vi "Topmost VI who Registers all Errors.vi"() -> ()   [LabVIEW 2017]
uses:
  user.lib/_NEVSTOP/Communicable State Machine(CSM)/AdvanceAPI/CSM - Make String Arguments Safe.vi
  user.lib/_NEVSTOP/Communicable State Machine(CSM)/AdvanceAPI/CSM - Break Down Multiple States String.vi
  user.lib/_NEVSTOP/Communicable State Machine(CSM)/AdvanceAPI/CSM - Compact Multiple States.vi
  user.lib/_NEVSTOP/Communicable State Machine(CSM)/AdvanceAPI/CSM - Keywords.vi
  user.lib/_NEVSTOP/Communicable State Machine(CSM)/Communicable State Machine.lvlib
panel:
  out "State History":string
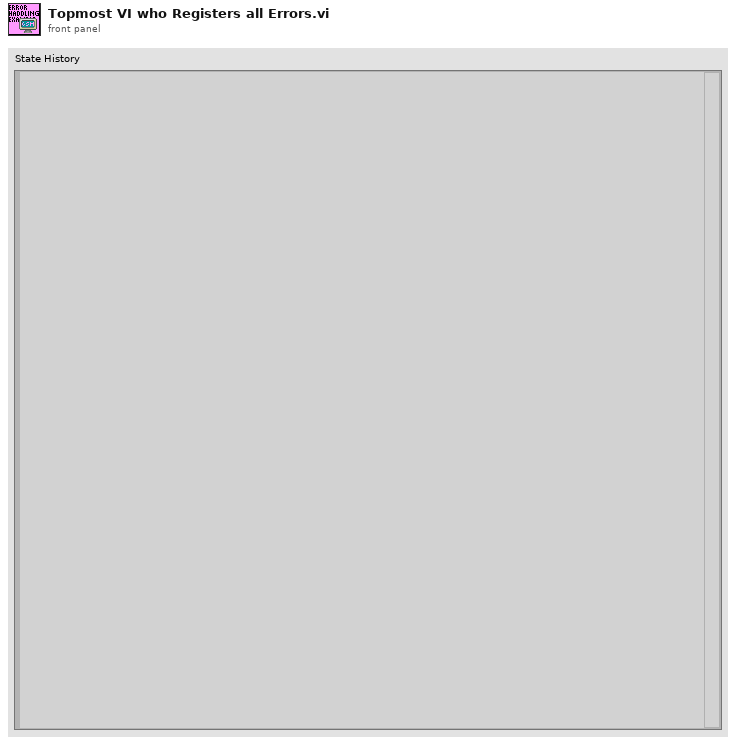
[diagram p1: front panel]
types:
  T1 = enum32{"Invalid", "Standard", "Closed", "Hidden", "Minimized", "Maximized"}
  T2 = enum32{"invalid app kind", "Development System", "Run Time System", "Student Edition", "Embedded LabVIEW", "Evaluation", "Custom"}
  T3 = typedef "Communicable State Machine.lvlib/_CSM_Response Source Message.ctl" = cluster{"‘State":string, "’Arguments":string, "’Error":errorcluster}
  T4 = cluster{"Current VI Reference":refnum<vi>, "Close Panel on Exit?":bool}
  T5 = cluster{"Core":cluster{"Current VI Reference":refnum<vi>, "Close Panel on Exit?":bool}, "Your Boolean data":bool, "Your string data":string}
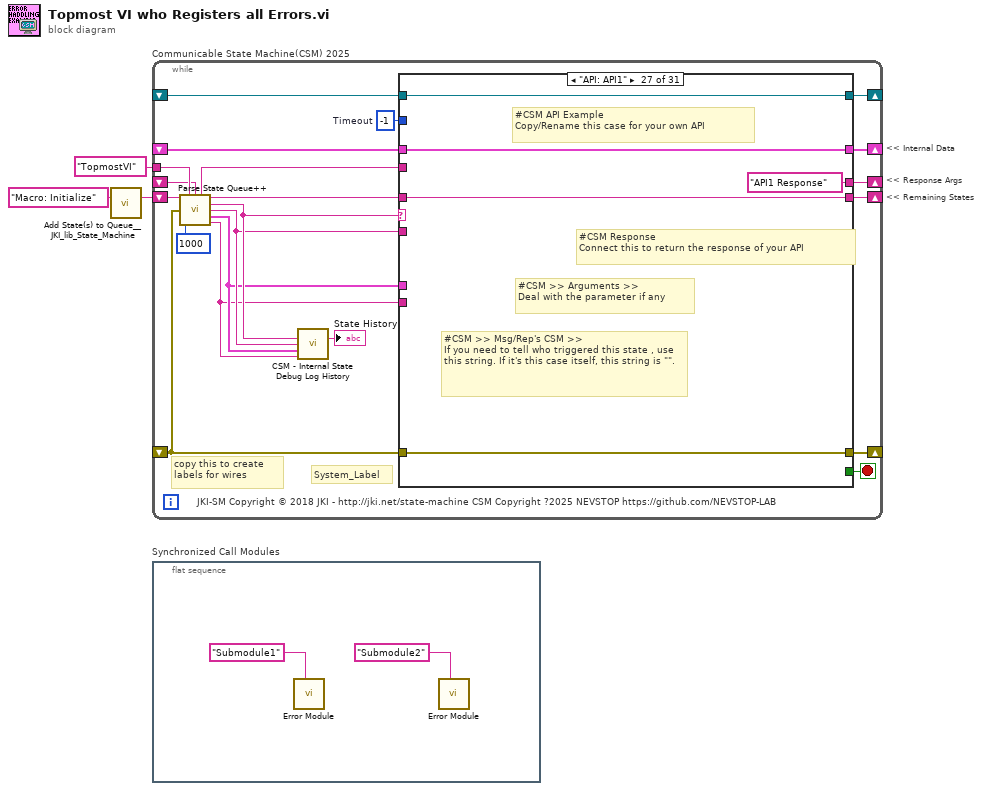
[diagram p0: block diagram]
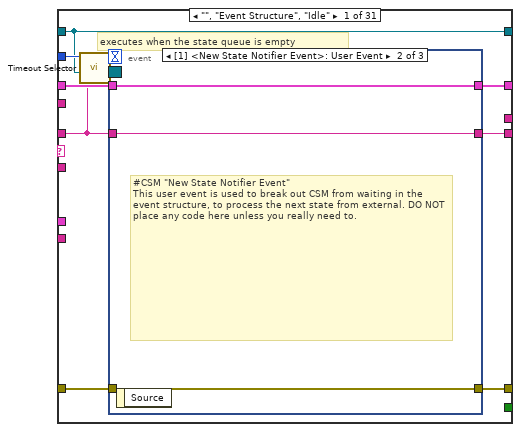
[diagram p2: hidden frame]
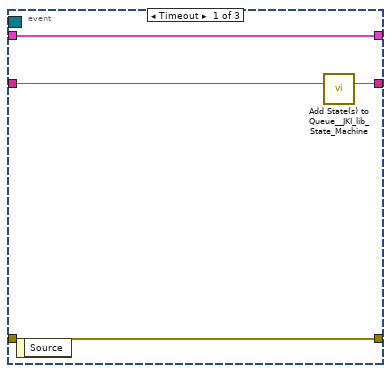
[diagram p3: hidden frame]
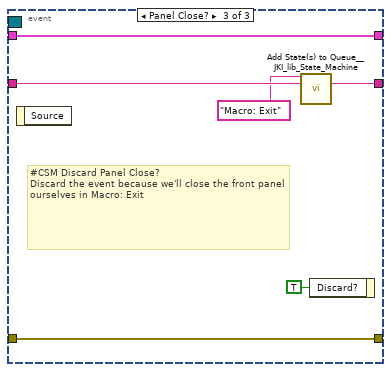
[diagram p4: hidden frame]
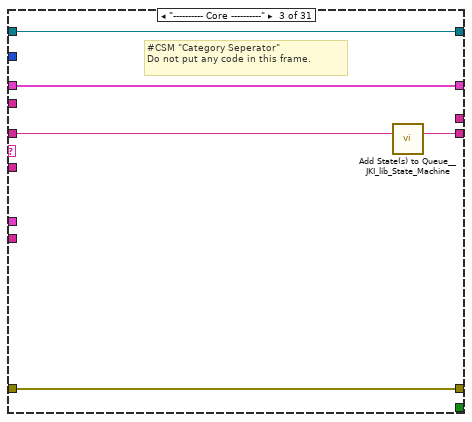
[diagram p6: hidden frame]
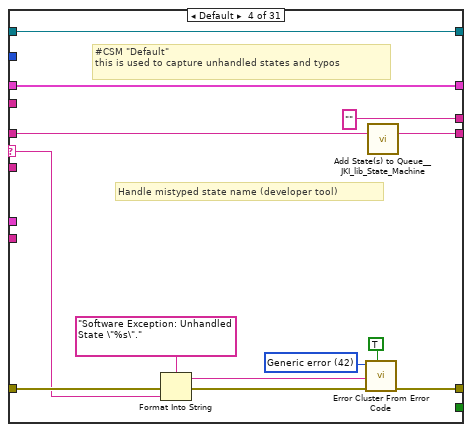
[diagram p7: hidden frame]
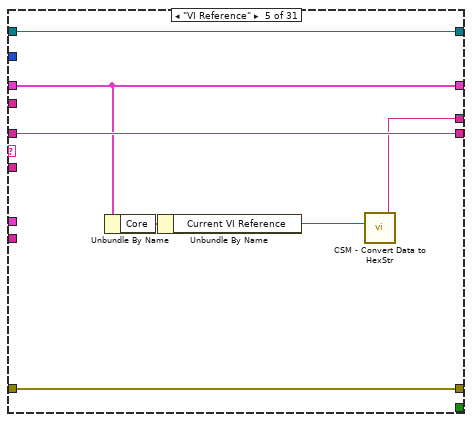
[diagram p8: hidden frame]
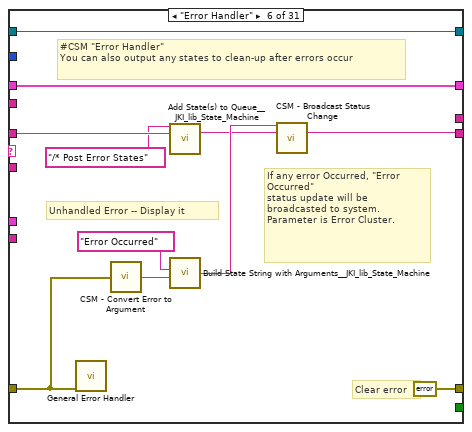
[diagram p9: hidden frame]
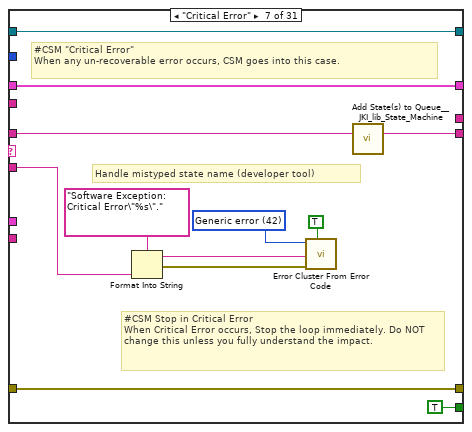
[diagram p10: hidden frame]
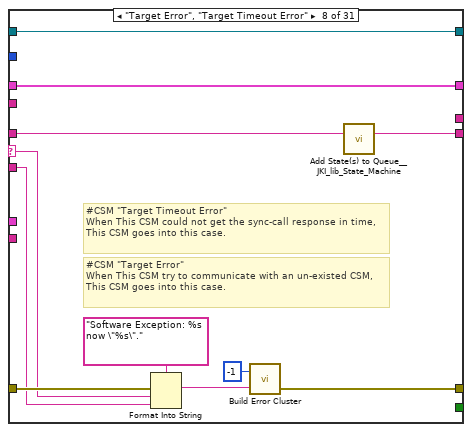
[diagram p11: hidden frame]
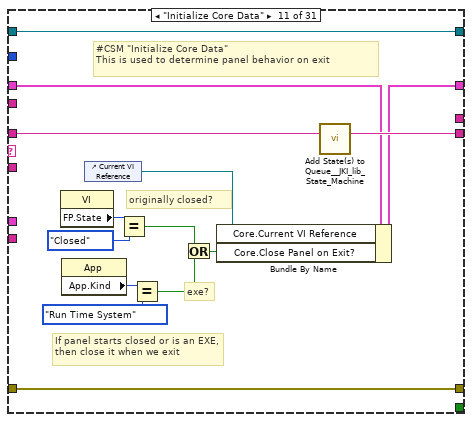
[diagram p14: hidden frame]
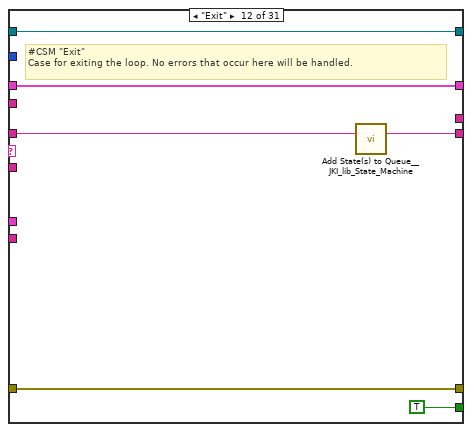
[diagram p15: hidden frame]
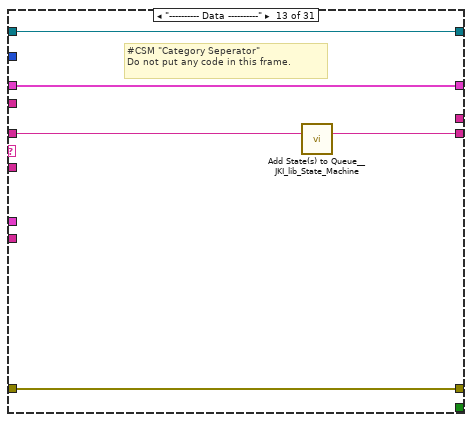
[diagram p16: hidden frame]
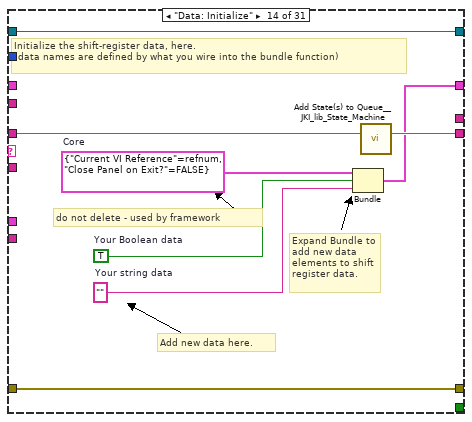
[diagram p17: hidden frame]
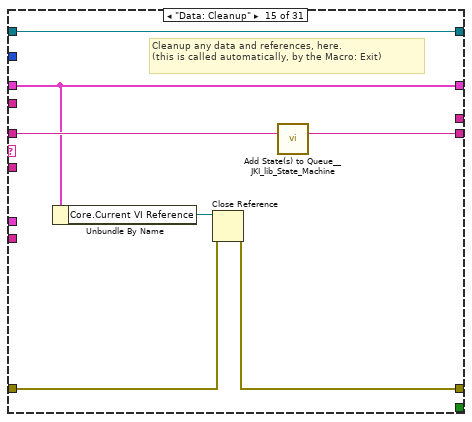
[diagram p18: hidden frame]
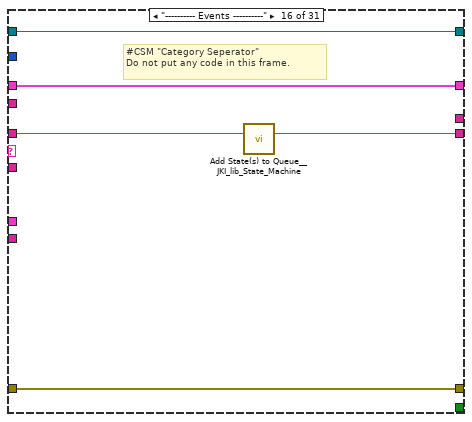
[diagram p19: hidden frame]
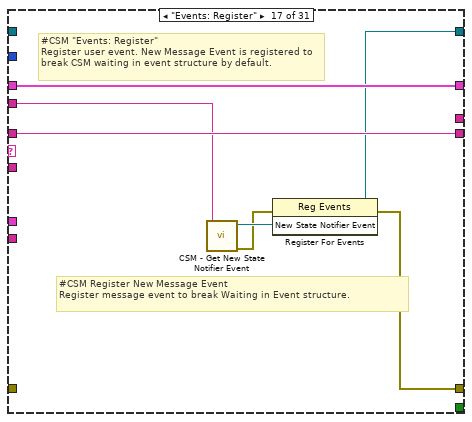
[diagram p20: hidden frame]
diagram:
  # "<< Internal Data"
  # "<< Response Args"
  # "<< Remaining States"
  n1 = call <vilib>:"Add State(s) to Queue__JKI_lib_State_Machine.vi"("State(s) in (\"\")"="Macro: Initialize") -> ("States Out"=w1:string)  [unwired: 14 in]
  n2 = while "Communicable State Machine(CSM) 2025" {
    shift-right: [w19] -> _
    shift-left: _ -> [w18]
    shift-right: [w22] -> _
    shift-left: _ -> [w16]
    shift-right: [w21] -> _
    shift-left: w1 -> [w23]
    tunnel: "TopmostVI" ("Name(\"\" to use uuid)") -> [w11]
    shift-right: [w14] -> _
    shift-left: _ -> [w5]
    shift-right: [w13] -> _
    shift-left: _ -> [w12]
    stop <- w20 stop-if-true
    w17 = -1  # Timeout
    # "copy this to create labels for wires"
    # "System_Label"
    # "JKI-SM Copyright © 2018 JKI - http://jki.net/state-machine CSM Copyright ?2025 NEVSTOP https://github.com/NEVSTOP-LAB"
    n3 = call "Parse State Queue++.vi"("State Queue"=w23, "Name(\"\" to use uuid)"=w11, "Response Arguments"=w5, "Previous Error"=w16, "Response Timeout(-2 use global Settings)"=1000 ("Response Timeout(1000ms)")) -> ("Name Used"=w6:string, "Remaining States"=w24:string, "Current State"=w10:string, "Arguments"=w9:string, ">> Response Source Message >>"=w8:T3, ">> Source CSM >>"=w7:string)  [unwired: 5 in]
    n4 = call "CSM - Internal State Debug Log History.vi"("State"=w10, "Arguments (\"\")"=w9, ">> Response Source Message >>"=w8, "Source (\"\")"=w7) -> ("Debug Log"=→"State History":string)  [unwired: 11 in]
    n5 = case shown="\"API: API1\"" w10 {
      selector: w10 -> [_ _ _ w58 _ _ _ w102 _ _ _ _ _ _ _ _ _ _ _ _ _ _ _ _ _ _ _ _ _ _ _]
      tunnel: w24 -> [w25 w49 w55 w62 w74 w86 w96 w104 w112 w116 w131 w137 w142 w150 w157 w162 w169 w173 w179 w184 w191 w207 w277 w283 w295 w298 w303 w309 w317 w323 w329]
      tunnel: w9 -> [_ _ _ _ _ _ w89 w103 _ _ _ _ _ _ _ _ _ _ _ _ w186 w201 _ _ _ _ _ w306 _ _ _]
      tunnel: w18 -> [w32 w48 w52 w60 w73 w84 w97 w106 w111 w115 w124 w135 w139 _ w152 w159 w168 w172 w176 w182 w189 w203 w274 w280 w292 w297 w302 w308 w314 w320 w326]
      tunnel: [w31 w50 w53 w64 w75 errorcluster {"status"=FALSE, "code"=0, "source"=""} ("error out") w98 w100 w113 w117 w128 w134 w140 w147 w153 w160 w163 w171 w177 w181 w187 w204 w275 w281 w293 w299 w304 w310 w315 w321 w327] -> w22
      tunnel: w16 -> [w30 w50 w53 w63 w75 w76 w98 w108 w113 w117 w128 w134 w140 w147 w154 w160 _ w174 w177 w181 w188 w205 w275 w281 w293 w299 w304 w310 w315 w321 w327]
      tunnel: [w33 w49 w54 w61 w74 w77 w95 w107 w112 w116 w130 w136 w141 w149 w156 w161 w169 w173 w178 w183 w190 w206 w276 w282 w294 w298 w303 w309 w316 w322 w328] -> w21
      tunnel: [_ _ _ _ _ _ TRUE _ _ _ _ TRUE _ _ _ _ _ _ _ _ _ _ _ _ _ _ _ _ _ _ _] -> w20
      tunnel: [w29 w48 w52 w60 w73 w84 w97 w106 w111 w115 w129 w135 w139 w148 w152 w159 w168 w172 w176 w182 w189 w203 w274 w280 w292 w297 w302 w308 w314 w320 w326] -> w19
      tunnel: w17 -> [w28 _ _ _ _ _ _ _ _ _ _ _ _ _ _ _ _ _ _ _ _ _ _ _ _ _ _ _ _ _ _]
      tunnel: w7 -> [_ _ _ _ _ _ _ _ _ _ _ _ _ _ _ _ _ _ _ _ _ _ _ _ _ _ _ _ _ _ _]
      tunnel: w8 -> [_ _ _ _ _ _ _ _ _ _ _ _ _ _ _ _ _ _ _ _ _ _ _ _ _ _ _ _ _ _ _]
      tunnel: [_ _ _ "" w69 _ _ _ _ _ _ _ _ _ _ _ _ _ _ _ _ _ _ _ _ _ "API1 Response" w305 _ "DoA Finished" "DoB Finished"] -> w14
      tunnel: [w27 w47 w51 w56 w72 w82 w87 w105 w110 w114 w118 w132 w138 w143 w151 w158 w167 w170 w175 w180 w185 w200 w273 w278 w285 w296 w301 w307 w313 w319 w325] -> w13
      tunnel: w12 -> [w27 w47 w51 w56 w72 w82 w87 w105 w110 w114 w118 w132 w138 w143 w151 w158 _ w170 w175 w180 w185 w200 w273 w278 w285 w296 w301 w307 w313 w319 w325]
      tunnel: w6 -> [_ _ _ _ _ _ _ _ _ _ _ _ _ _ _ _ w166 _ _ _ _ _ _ _ _ _ _ _ _ _ _]
      frame "", "Event Structure", "Idle" {
        # "executes when the state queue is empty"
        n6 = call "Timeout Selector.vi"("Remaining States"=w25, "Timeout Expected"=w28) -> ("Timeout"=w26:i32)  [unwired: 5 in]
        n7 = event shown="[1] <New State Notifier Event>: User Event" {
          selector: w27 -> [_ _ _]
          dyn-events: _ -> [_ _ _]
          timeout: w26 -> [_ _ _]
          tunnel: w25 -> [w37 w39 w46]
          tunnel: [w36 w39 w45] -> w33
          tunnel: w32 -> [w34 w40 w43]
          tunnel: [w35 w38 w44] -> w31
          tunnel: w30 -> [w35 w38 w44]
          tunnel: [w34 w40 w43] -> w29
          event Timeout {
            n8 = event-data() -> ()  [unwired: 1 in, 1 out]
            n9 = call <vilib>:"Add State(s) to Queue__JKI_lib_State_Machine.vi"("State(s) in (\"\")"=w37) -> ("States Out"=w36:string)  [unwired: 14 in]
          }
          event User Event {
            # "#CSM \"New State Notifier Event\"\nThis user event is used to break out CSM from waiting in the event structure, to process the next state from external. DO NOT place any code here unless you really need to."
            n10 = event-data() -> ()  [unwired: 1 in, 1 out]
          }
          event Panel Close? {
            # "#CSM Discard Panel Close?\nDiscard the event because we'll close the front panel ourselves in Macro: Exit"
            n11 = event-data() -> ()  [unwired: 1 in, 1 out]
            n12 = call <vilib>:"Add State(s) to Queue__JKI_lib_State_Machine.vi"("State(s) in Front (\"\")"="Macro: Exit", "State(s) in (\"\")"=w46) -> ("States Out"=w45:string)  [unwired: 13 in]
            n13 = event-data("Discard?"=TRUE) -> ()  [unwired: 1 in, 1 out]
          }
        }
      }
      frame "CSM Documentation" {
        # "#CSM README FIRST\n\nCSM is a LabVIEW application framework that builds upon JKI State Machine (JKISM). It follows the pattern of JKISM and extends the keywords to describe message communication between CSM modules, including concepts such as Sync-Message, Async-Message, Subscription/Unsubscription of status - essential elements for creating reusable code modules. For more information, please visit the CSM wiki: https://github.com/NEVSTOP-LAB/JKI-State-Machine-Plus-Plus/wiki\n\nFor instructions on JKI State Machine, visit: http://jki.net/state-machine/\nFor information about CSM, visit: https://github.com/NEVSTOP-LAB"
        # "#CSM \"Documentation\"\nCase for holding CSM Documenation"
      }
      frame "---------- Core ----------" {
        # "#CSM \"Category Seperator\"\nDo not put any code in this frame."
        n14 = call <vilib>:"Add State(s) to Queue__JKI_lib_State_Machine.vi"("State(s) in (\"\")"=w55) -> ("States Out"=w54:string)  [unwired: 14 in]
      }
      frame Default {
        w67 = 42 items=["No error", "Argument error", "Memory is full", "Out of zone", "End of file", "File already open", "Generic file I/O error", "File not found", "File permission error", "Disk is full", "Duplicate path", "Too many files open", "System feature not enabled", "Resource file not found", "Cannot add resource", "Resource not found", "Image not found", "Image memory error", "Pen does not exist", "Config type invalid", "Config token not found", "Config parse error", "Config memory error", "Bad external code format", "Bad external code offset", "External code not present", "Null window", "Destroy window error", "Null menu", "Print aborted", "Bad print record", "Print driver error", "Windows error during printing", "Memory error during printing", "Print dialog error", "Generic print error", "Invalid device refnum", "Device not found", "Device parameter error", "Device unit error", "Cannot open device", "Device call aborted", "Generic error", "Cancelled by user", "Object ID too low", "Object ID too high", "Object not in heap", "Unknown heap", "Unknown object (invalid DefProc)", "Unknown object (DefProc not in table)", "Message out of range", "Invalid (null) method", "Unknown message", "Manager call not supported", "Bad address", "Network operation in progress", "Network operation timed out", "Connection is busy", "Network attribute not supported", "Network error", "Address in use", "System out of memory", "Connection aborted", "Connection refused", "Not connected", "Already connected", "Connection closed", "Initialization error (interapplication manager)", "Bad occurrence", "Wait on unbound occurrence handler", "Occurrence queue overflow", "Datalog type conflict", "Unused", "Unrecognized type (interapplication manager)", "Memory corrupt", "Failed to make temporary DLL", "Old CIN version", "Drag socket not found", "Failed to load drop-object", "Failed to register OLE object", "Failed to release OLE object", "Format specifier type mismatch", "Unknown format specifier", "Too few format specifiers", "Too many format specifiers", "Scan failed", "Newer CIN version", "Error converting to variant", "Runtime menu error", "Password tampered", "Variant attribute not found", "Incompatible variant data type", "Event data is not available", "Event Store is not present", "Occurrence is not found", "Event Queue is not created", "Event info is not available", "Refnum passed is NULL", "Error retrieving Class GUID", "Error retrieving CoClass GUID", "Error retrieving TypeLib GUID.", "Bad built application magic bytes.", "Specific driver is different from the specific driver associated with the Logical Name.", "There is no session opened to the class driver.", "Max Error", "MAX - Error with config objects", "MAX - Error loading configuration", "MAX - Group not supported"]
        # "#CSM \"Default\"\nthis is used to capture unhandled states and typos"
        # "Handle mistyped state name (developer tool)"
        n15 = Format Into String(format string="Software Exception: Unhandled State \"%s\"." ("message"), error in=w63, w58) -> (resulting string=w66:string, error out=w65:errorcluster)  [unwired: 1 in]
        n16 = call <vilib>:"Error Cluster From Error Code.vi"("show call chain? (False)"=TRUE, "error in (no error)"=w65, "error message (\"\")"=w66, "error code (0)"=w67) -> ("error out"=w64:errorcluster)  [unwired: 5 in]
        n17 = call <vilib>:"Add State(s) to Queue__JKI_lib_State_Machine.vi"("State(s) in (\"\")"=w62) -> ("States Out"=w61:string)  [unwired: 14 in]
      }
      frame "VI Reference" {
        n18 = Unbundle By Name(w73) -> ("Core"=w71:T4)
        n19 = Unbundle By Name(w71) -> ("Current VI Reference"=w70:refnum<vi>)
        n20 = call "CSM - Convert Data to HexStr.vi"("Variant"=w70) -> ("HEX String (0-9,A-F)"=w69:string)  [unwired: 8 in]
      }
      frame "Error Handler" {
        # "#CSM \"Error Handler\"\nYou can also output any states to clean-up after errors occur"
        # "If any error Occurred, \"Error Occurred\" \nstatus update will be broadcasted to system.\nParameter is Error Cluster."
        # "Unhandled Error -- Display it"
        # "Clear error"
        n21 = call <vilib>:"General Error Handler.vi"("error in (no error)"=w76) -> ()  [unwired: 10 in, 5 out]
        n22 = call "CSM - Convert Error to Argument.vi"("error"=w76) -> ("Argument"=w80:string)  [unwired: 4 in]
        n23 = call <vilib>:"Add State(s) to Queue__JKI_lib_State_Machine.vi"("State(s) in Front (\"\")"="/* Post Error States", "State(s) in (\"\")"=w86) -> ("States Out"=w78:string)  [unwired: 13 in]
        n24 = call <vilib>:"Build State String with Arguments__JKI_lib_State_Machine.vi"("Arguments (\"\")"=w80, "State"="Error Occurred" ("Status with Arguments")) -> ("State with Arguments"=w79:string)  [unwired: 4 in]
        n25 = call "CSM - Broadcast Status Change.vi"("Status with Arguments"=w79, "State Queue"=w78) -> ("Remaining States"=w77:string)  [unwired: 13 in]
      }
      frame "Critical Error" {
        w93 = 42 items=["No error", "Argument error", "Memory is full", "Out of zone", "End of file", "File already open", "Generic file I/O error", "File not found", "File permission error", "Disk is full", "Duplicate path", "Too many files open", "System feature not enabled", "Resource file not found", "Cannot add resource", "Resource not found", "Image not found", "Image memory error", "Pen does not exist", "Config type invalid", "Config token not found", "Config parse error", "Config memory error", "Bad external code format", "Bad external code offset", "External code not present", "Null window", "Destroy window error", "Null menu", "Print aborted", "Bad print record", "Print driver error", "Windows error during printing", "Memory error during printing", "Print dialog error", "Generic print error", "Invalid device refnum", "Device not found", "Device parameter error", "Device unit error", "Cannot open device", "Device call aborted", "Generic error", "Cancelled by user", "Object ID too low", "Object ID too high", "Object not in heap", "Unknown heap", "Unknown object (invalid DefProc)", "Unknown object (DefProc not in table)", "Message out of range", "Invalid (null) method", "Unknown message", "Manager call not supported", "Bad address", "Network operation in progress", "Network operation timed out", "Connection is busy", "Network attribute not supported", "Network error", "Address in use", "System out of memory", "Connection aborted", "Connection refused", "Not connected", "Already connected", "Connection closed", "Initialization error (interapplication manager)", "Bad occurrence", "Wait on unbound occurrence handler", "Occurrence queue overflow", "Datalog type conflict", "Unused", "Unrecognized type (interapplication manager)", "Memory corrupt", "Failed to make temporary DLL", "Old CIN version", "Drag socket not found", "Failed to load drop-object", "Failed to register OLE object", "Failed to release OLE object", "Format specifier type mismatch", "Unknown format specifier", "Too few format specifiers", "Too many format specifiers", "Scan failed", "Newer CIN version", "Error converting to variant", "Runtime menu error", "Password tampered", "Variant attribute not found", "Incompatible variant data type", "Event data is not available", "Event Store is not present", "Occurrence is not found", "Event Queue is not created", "Event info is not available", "Refnum passed is NULL", "Error retrieving Class GUID", "Error retrieving CoClass GUID", "Error retrieving TypeLib GUID.", "Bad built application magic bytes.", "Specific driver is different from the specific driver associated with the Logical Name.", "There is no session opened to the class driver.", "Max Error", "MAX - Error with config objects", "MAX - Error loading configuration", "MAX - Group not supported"]
        # "#CSM Stop in Critical Error\nWhen Critical Error occurs, Stop the loop immediately. Do NOT change this unless you fully understand the impact."
        # "#CSM \"Critical Error\"\nWhen any un-recoverable error occurs, CSM goes into this case."
        # "Handle mistyped state name (developer tool)"
        n26 = Format Into String(format string="Software Exception: Critical Error\"%s\"." ("message"), w89) -> (resulting string=w92:string, error out=w91:errorcluster)  [unwired: 2 in]
        n27 = call <vilib>:"Error Cluster From Error Code.vi"("show call chain? (False)"=TRUE, "error in (no error)"=w91, "error message (\"\")"=w92, "error code (0)"=w93) -> ()  [unwired: 5 in, 1 out]
        n28 = call <vilib>:"Add State(s) to Queue__JKI_lib_State_Machine.vi"("State(s) in (\"\")"=w96) -> ("States Out"=w95:string)  [unwired: 14 in]
      }
      frame "Target Error", "Target Timeout Error" {
        # "#CSM \"Target Error\"\nWhen This CSM try to communicate with an un-existed CSM, This CSM goes into this case."
        # "#CSM \"Target Timeout Error\"\nWhen This CSM could not get the sync-call response in time, This CSM goes into this case."
        n29 = Format Into String(format string="Software Exception: %s now \"%s\"." ("message"), error in=w108, w102, w103) -> (resulting string=w101:string)  [unwired: 1 in, 1 out]
        n30 = call "Build Error Cluster.vi"("String to Prepend to source (\"\")"=w101, "code"=-1) -> ("error out"=w100:errorcluster)
        n31 = call <vilib>:"Add State(s) to Queue__JKI_lib_State_Machine.vi"("State(s) in (\"\")"=w104) -> ("States Out"=w107:string)  [unwired: 14 in]
      }
      frame "Async Response", "Response" {
        # "#CSM Response Comments\nAfter Message is executed, CSM goes to this state for receive the response.\n    For Async Message(->), \"Async Response\" is used. This CSM will goes to \"Async Message Posted\" immediately and receive the \"Async Response\" after the callee finishes the message.\n    For Sync Message(@),  This CSM will wait until the message is done and immediately goes to \"Response\""
        # "#CSM \"Async Response\"\nHandle Async-call Response (\"Async Response\" for ->)"
        # "#CSM \"Response\"\nHandle Sync-call Response (\"Response\" for -@)"
      }
      frame "Async Message Posted" {
        # "#CSM \"Async Message Posted\"\nAfter Async Message is posted (-> or ->| ), CSM goes to this state for post-action.\nYou can use Argument - State to tell which Async Message is called."
      }
      frame "Initialize Core Data" {
        # "#CSM \"Initialize Core Data\"\nThis is used to determine panel behavior on exit"
        # "originally closed?"
        # "exe?"
        # "If panel starts closed or is an EXE, then close it when we exit"
        n32 = property class="VI"() -> ("FP.State"=w121:T1)  [unwired: 2 in, 2 out]
        n33 = property class="App"() -> ("App.Kind"=w127:T2)  [unwired: 2 in, 2 out]
        n34 = control-ref of="Current VI Reference"() -> (w122:refnum<vi>)
        n35 = Equal?(x=w121, y=T1."Closed" ("Front Panel Window:State")) -> (x = y?=w119:bool)
        n36 = Equal?(x=w127, y=T2."Run Time System" ("Application:Kind")) -> (x = y?=w125:bool)
        n37 = Or(x=w119, y=w125) -> (x .or. y?=w123:bool)
        n38 = Bundle By Name(cluster=w124, "Core.Current VI Reference"=w122, "Core.Close Panel on Exit?"=w123) -> (w129:T5)
        n39 = call <vilib>:"Add State(s) to Queue__JKI_lib_State_Machine.vi"("State(s) in (\"\")"=w131) -> ("States Out"=w130:string)  [unwired: 14 in]
      }
      frame "Exit" {
        # "#CSM \"Exit\"\nCase for exiting the loop. No errors that occur here will be handled."
        n40 = call <vilib>:"Add State(s) to Queue__JKI_lib_State_Machine.vi"("State(s) in (\"\")"=w137) -> ("States Out"=w136:string)  [unwired: 14 in]
      }
      frame "---------- Data ----------" {
        # "#CSM \"Category Seperator\"\nDo not put any code in this frame."
        n41 = call <vilib>:"Add State(s) to Queue__JKI_lib_State_Machine.vi"("State(s) in (\"\")"=w142) -> ("States Out"=w141:string)  [unwired: 14 in]
      }
      frame "Data: Initialize" {
        w144 = T4 {"Current VI Reference"=refnum, "Close Panel on Exit?"=FALSE}  # Core
        w146 = TRUE  # Your Boolean data
        w145 = ""  # Your string data
        # "do not delete - used by framework"
        # "Expand Bundle to add new data elements to shift register data."
        # "Add new data here."
        # "Initialize the shift-register data, here.\n(data names are defined by what you wire into the bundle function)"
        n42 = Bundle("Core"=w144, "Your Boolean data"=w146, "Your string data"=w145) -> (w148:T5)  [unwired: 1 in]
        n43 = call <vilib>:"Add State(s) to Queue__JKI_lib_State_Machine.vi"("State(s) in (\"\")"=w150) -> ("States Out"=w149:string)  [unwired: 14 in]
      }
      frame "Data: Cleanup" {
        # "Cleanup any data and references, here.\n(this is called automatically, by the Macro: Exit)"
        n44 = Unbundle By Name(w152) -> ("Core.Current VI Reference"=w155:refnum<vi>)
        n45 = Close Reference(reference=w155, error in (no error)=w154) -> (error out=w153:errorcluster)
        n46 = call <vilib>:"Add State(s) to Queue__JKI_lib_State_Machine.vi"("State(s) in (\"\")"=w157) -> ("States Out"=w156:string)  [unwired: 14 in]
      }
      frame "---------- Events ----------" {
        # "#CSM \"Category Seperator\"\nDo not put any code in this frame."
        n47 = call <vilib>:"Add State(s) to Queue__JKI_lib_State_Machine.vi"("State(s) in (\"\")"=w162) -> ("States Out"=w161:string)  [unwired: 14 in]
      }
      frame "Events: Register" {
        # "#CSM \"Events: Register\"\nRegister user event. New Message Event is registered to break CSM waiting in event structure by default."
        # "#CSM Register New Message Event\nRegister message event to break Waiting in Event structure."
        n48 = call "CSM - Get New State Notifier Event.vi"("Name(\"\" to use uuid) in"=w166) -> ("Error out"=w164:errorcluster, "New State Notifier Event"=w165:refnum<user-event>)  [unwired: 9 in]
        n49 = register-events(error in=w164, w165) -> (reference out=w167:refnum<event-registration>, error out=w163:errorcluster)  [unwired: 1 in]
      }
      frame "Events: Unregister" {
        # "#CSM \"Events: Unregister\"\nUnregister user event."
        n50 = Unregister For Events(event registration refnum=w170, error in=w174) -> (error out=w171:errorcluster)
      }
      frame "---------- UI ----------" {
        # "#CSM \"Category Seperator\"\nDo not put any code in this frame."
        n51 = call <vilib>:"Add State(s) to Queue__JKI_lib_State_Machine.vi"("State(s) in (\"\")"=w179) -> ("States Out"=w178:string)  [unwired: 14 in]
      }
      frame "UI: Initialize" {
        # "#CSM \"UI: Initialize\"\nInitialize the User Interface, here.\n(this is called automatically, by the Macro: Init)"
        n52 = call <vilib>:"Add State(s) to Queue__JKI_lib_State_Machine.vi"("State(s) in (\"\")"=w184) -> ("States Out"=w183:string)  [unwired: 14 in]
      }
      frame "UI: Cursor Set" {
        # "#CSM \"UI: Cursor Set\"\nSet and Unset Cursor Busy.\n(Usage: \"UI: Cursor Set >> Busy|Idle\")"
        # "Argument"
        n53 = disable-structure shown="TARGET_TYPE!=Windows" {
          disable-tunnel: w188 -> [w194 w199]
          disable-tunnel: [w193 w199] -> w187
          disable-tunnel: w186 -> [w192 _]
          frame condition #0 (active) {
            n54 = case shown="\"Idle\", Default" w192 {
              tunnel: w194 -> [w196 w198]
              tunnel: [w195 w197] -> w193
              frame "Idle", Default {
                n55 = call <vilib>:"Unset Busy.vi"("error in (no error)"=w196) -> ("error out"=w195:errorcluster)  [unwired: 10 in]
              }
              frame "Busy" {
                n56 = call <vilib>:"Set Busy.vi"("error in (no error)"=w198) -> ("error out"=w197:errorcluster)  [unwired: 9 in, 1 out]
              }
            }
          }
          frame condition #1 {
          }
        }
        n57 = call <vilib>:"Add State(s) to Queue__JKI_lib_State_Machine.vi"("State(s) in (\"\")"=w191) -> ("States Out"=w190:string)  [unwired: 14 in]
      }
      frame "UI: Front Panel State" {
        # "#CSM \"UI: Front Panel State\"\nSet Front Panel Open or Closed\n(Usage: \"UI: Front Panel State >> Open|Close\")"
        # "Argument"
        n58 = Unbundle By Name(w203) -> ("Core.Current VI Reference"=w202:refnum<vi>)
        n59 = call <vilib>:"Add State(s) to Queue__JKI_lib_State_Machine.vi"("State(s) in (\"\")"=w207) -> ("States Out"=w206:string)  [unwired: 14 in]
        n60 = case shown="\"Close\", \"Closed\"" w201 {
          tunnel: w205 -> [w213 w228 w239 w252 w265]
          tunnel: [w215 w229 w241 w254 w267] -> w204
          tunnel: w202 -> [w214 w226 w240 w253 w266]
          frame "Open", "Standard", Default {
            w208 = T1."Standard" ("State")
            n61 = property class="VI"(reference=w214, error in=w213) -> (reference out=w211:refnum<vi>, error out=w212:errorcluster, "FP.State"=w210:T1)
            n62 = Not Equal?(x=w210, y=w208) -> (x != y?=w209:bool)
            n63 = case shown="True" w209 {
              tunnel: [w219 w221] -> w215
              tunnel: w212 -> [w218 w221]
              tunnel: w211 -> [w217 _]
              tunnel: w208 -> [w216 _]
              frame True {
                n64 = invoke class="VI" method="FP.Open"(reference=w217, error in=w218, "Activate"=TRUE, "State"=w216) -> (error out=w219:errorcluster)  [unwired: 1 in, 4 out]
              }
              frame False {
              }
            }
          }
          frame "Close", "Closed" {
            n65 = property class="VI"(reference=w226, error in=w228) -> (reference out=w225:refnum<vi>, error out=w227:errorcluster, "FP.State"=w223:T1)
            n66 = Not Equal?(x=w223, y=T1."Closed" ("Front Panel Window:State")) -> (x != y?=w222:bool)
            n67 = case shown="False" w222 {
              tunnel: [w230 w233] -> w229
              tunnel: w227 -> [w230 w232]
              tunnel: w225 -> [_ w231]
              frame False {
              }
              frame True {
                n68 = invoke class="VI" method="FP.Close"(reference=w231, error in=w232) -> (error out=w233:errorcluster)  [unwired: 1 in, 2 out]
              }
            }
          }
          frame "Hidden", "Hide" {
            w234 = T1."Hidden" ("State")
            n69 = property class="VI"(reference=w240, error in=w239) -> (reference out=w237:refnum<vi>, error out=w238:errorcluster, "FP.State"=w236:T1)
            n70 = Not Equal?(x=w236, y=w234) -> (x != y?=w235:bool)
            n71 = case shown="True" w235 {
              tunnel: [w245 w246] -> w241
              tunnel: w238 -> [w244 w246]
              tunnel: w237 -> [w243 _]
              tunnel: w234 -> [w242 _]
              frame True {
                n72 = invoke class="VI" method="FP.Open"(reference=w243, error in=w244, "State"=w242) -> (error out=w245:errorcluster)  [unwired: 2 in, 4 out]
              }
              frame False {
              }
            }
          }
          frame "Minimize", "Minimized" {
            w247 = T1."Minimized" ("State")
            n73 = property class="VI"(reference=w253, error in=w252) -> (reference out=w250:refnum<vi>, error out=w251:errorcluster, "FP.State"=w249:T1)
            n74 = Not Equal?(x=w249, y=w247) -> (x != y?=w248:bool)
            n75 = case shown="True" w248 {
              tunnel: [w258 w259] -> w254
              tunnel: w251 -> [w257 w259]
              tunnel: w250 -> [w256 _]
              tunnel: w247 -> [w255 _]
              frame True {
                n76 = invoke class="VI" method="FP.Open"(reference=w256, error in=w257, "State"=w255) -> (error out=w258:errorcluster)  [unwired: 2 in, 4 out]
              }
              frame False {
              }
            }
          }
          frame "Maximize", "Maximized" {
            w260 = T1."Maximized" ("State")
            n77 = property class="VI"(reference=w266, error in=w265) -> (reference out=w263:refnum<vi>, error out=w264:errorcluster, "FP.State"=w262:T1)
            n78 = Not Equal?(x=w262, y=w260) -> (x != y?=w261:bool)
            n79 = case shown="True" w261 {
              tunnel: [w271 w272] -> w267
              tunnel: w264 -> [w270 w272]
              tunnel: w263 -> [w269 _]
              tunnel: w260 -> [w268 _]
              frame True {
                n80 = invoke class="VI" method="FP.Open"(reference=w269, error in=w270, "State"=w268) -> (error out=w271:errorcluster)  [unwired: 2 in, 4 out]
              }
              frame False {
              }
            }
          }
        }
      }
      frame "---------- Macro ----------" {
        # "#CSM \"Category Seperator\"\nDo not put any code in this frame."
        n81 = call <vilib>:"Add State(s) to Queue__JKI_lib_State_Machine.vi"("State(s) in (\"\")"=w277) -> ("States Out"=w276:string)  [unwired: 14 in]
      }
      frame "Macro: Initialize" {
        w279 = "Data: Initialize\nInitialize Core Data\nEvents: Register\nUI: Initialize\nUI: Front Panel State >> Open\n\n//Reigster all Errors if you are topmost VI\nError Occurred@* >> Error Handler -><register>"  # Data: Initialize Initialize Core Data Events: Register UI: Initialize UI: Front Panel State >> Open  //Reigster all Errors if you are topmost VI Error Occurred@* >> Error Handler -><register>
        # "#CSM \"Macro: Initialize\"\nInitialization Macro (This is called once, when the VI starts)"
        n82 = call <vilib>:"Add State(s) to Queue__JKI_lib_State_Machine.vi"("State(s) in Front (\"\")"=w279, "State(s) in (\"\")"=w283) -> ("States Out"=w282:string)  [unwired: 13 in]
      }
      frame "Macro: Exit" {
        # "#CSM \"Macro: Exit\"\nExit Macro (This is called once, when the VI exits)"
        n83 = Unbundle By Name(w292) -> ("Core.Close Panel on Exit?"=w291:bool)
        n84 = Select(t="UI: Front Panel State >> Close", s=w291, f="") -> (s? t:f=w288:string)
        n85 = call <vilib>:"Add State(s) to Queue__JKI_lib_State_Machine.vi"("State(s) in Front (\"\")"="Macro: Exit -@ Submodule1\nMacro: Exit -@ Submodule2", "State(s) in (\"\")"=w288, "State(s) at Back (\"\")"="Data: Cleanup\nEvents: Unregister\nExit") -> ("States Out"=w286:string)  [unwired: 12 in]
        n86 = call <vilib>:"Add State(s) to Queue__JKI_lib_State_Machine.vi"("State(s) in Front (\"\")"=w286, "State(s) in (\"\")"=w295) -> ("States Out"=w294:string)  [unwired: 13 in]
      }
      frame "---------- API ----------" {
        # "#CSM \"Category Seperator\"\nDo not put any code in this frame."
      }
      frame "API: API1" {
        # "#CSM API Example\nCopy/Rename this case for your own API"
        # "#CSM Response\nConnect this to return the response of your API"
        # "#CSM >> Msg/Rep's CSM >>\nIf you need to tell who triggered this state , use this string. If it's this case itself, this string is \"\"."
        # "#CSM >> Arguments >>\nDeal with the parameter if any"
      }
      frame "API: API2" {
        # "#CSM API Example\nCopy/Rename this case for your own API"
        # "unpack Hex String  to Variant\nif complex parameter is needed."
        n87 = call "CSM - Convert HexStr to Data.vi"("HEX String"=w306) -> ()  [unwired: 7 in, 2 out]
        n88 = disable-structure shown="Disabled" {
          disable-tunnel: [w311 "API2 Response"] -> w305
          frame Disabled {
            # "pack variant to hexstr \nif complex response is needed."
            # "complex Response"
            n89 = call "CSM - Convert Data to HexStr.vi"() -> ("HEX String (0-9,A-F)"=w311:string)  [unwired: 9 in]
          }
          frame Enabled {
          }
        }
      }
      frame "---------- DoSth ----------" {
        # "#CSM \"Category Seperator\"\nDo not put any code in this frame."
        n90 = call <vilib>:"Add State(s) to Queue__JKI_lib_State_Machine.vi"("State(s) in (\"\")"=w317) -> ("States Out"=w316:string)  [unwired: 14 in]
      }
      frame "DoSth: DoA" {
        # "#CSM \"Internal State\"\nThis category is used for holding internal states"
        n91 = call <vilib>:"Add State(s) to Queue__JKI_lib_State_Machine.vi"("State(s) in (\"\")"=w323) -> ("States Out"=w322:string)  [unwired: 14 in]
      }
      frame "DoSth: DoB" {
        # "#CSM \"Internal State\"\nThis category is used for holding internal states"
        n92 = call <vilib>:"Add State(s) to Queue__JKI_lib_State_Machine.vi"("State(s) in (\"\")"=w329) -> ("States Out"=w328:string)  [unwired: 14 in]
      }
    }
  }
  n93 = flat-sequence "Synchronized Call Modules" {
    frame #0 {
      n94 = call "Error Module.vi"("Name(\"\" to use uuid)"="Submodule1" ("Name(\"\" to use uuid)")) -> ()  [unwired: 11 in]
      n95 = call "Error Module.vi"("Name(\"\" to use uuid)"="Submodule2" ("Name(\"\" to use uuid)")) -> ()  [unwired: 11 in]
    }
  }
